vi "parseModeFrame.vi"(8 "error in (no error)":errorcluster, 10 "ModbusBuffer in":refnum<class "ModbusBuffer.lvclass">, 11 "ILC in":refnum<class "ILC.lvclass">) -> (0 "error out":errorcluster, 2 "ModbusBuffer out":refnum<class "ModbusBuffer.lvclass">, 3 "ILC out":refnum<class "ILC.lvclass">)   [LabVIEW 2016, in "RTILC.lvlib" / "ILC.lvclass"]
uses:
  ILC.lvclass
  Common_RT_Modbus/ModbusBuffer/ModbusBuffer.lvclass
  Common_RT_Modbus/ModbusBuffer/ModbusBuffer.lvclass/ModbusBuffer.ctl
  Common_RT_Modbus/DataTypes/ExceptionCodes.ctl
  ILC.lvclass/ILC.ctl
  Common_RT_Modbus/ModbusBuffer/readU8.vi
  Common_RT_Modbus/ModbusBuffer/readTimestampByte.vi
  Common_RT_Modbus/ModbusBuffer/readInstructionByte.vi
  Common_RT_Modbus/RTModbus.lvlib
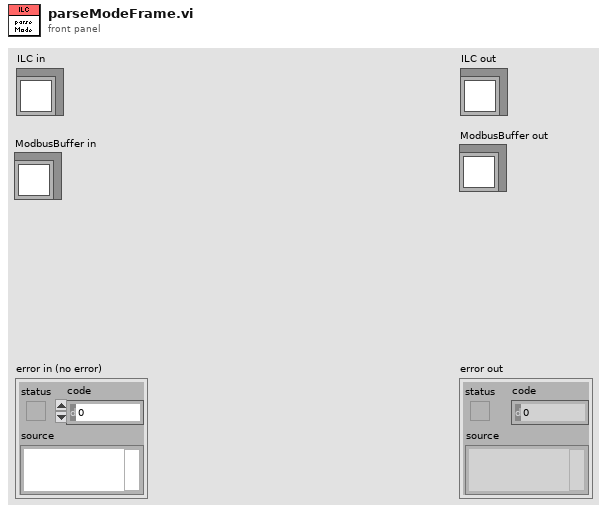
[diagram p1: front panel]
types:
  T1 = typedef "RTModbus.lvlib/ExceptionCodes.ctl" = u16
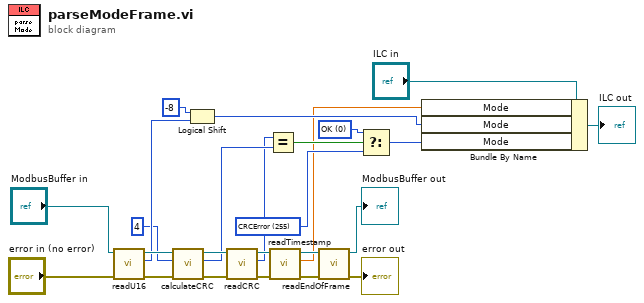
[diagram p0: block diagram]
diagram:
  w21 = T1 255 items=["OK"=0, "IllegalFunction"=1, "IllegalDataAddress"=2, "IllegalDataValue"=3, "SlaveDeviceFailure"=4, "Acknowledge"=5, "SlaveDeviceBusy"=6, "NegativeAcknowledge"=7, "MemoryParityError"=8, "GatewayPathUnavailable"=9, "GatewayTargetDeviceFailedToRespond"=10, "WaitingForResponse"=254, "CRCError"=255] ("f")
  w22 = T1 0 items=["OK"=0, "IllegalFunction"=1, "IllegalDataAddress"=2, "IllegalDataValue"=3, "SlaveDeviceFailure"=4, "Acknowledge"=5, "SlaveDeviceBusy"=6, "NegativeAcknowledge"=7, "MemoryParityError"=8, "GatewayPathUnavailable"=9, "GatewayTargetDeviceFailedToRespond"=10, "WaitingForResponse"=254, "CRCError"=255] ("Responses.ADCOffsetSensitivity")
  n1 = call "readU16.vi"("error in (no error)"="error in (no error)", "ModbusBuffer in"="ModbusBuffer in") -> ("error out"=w7:errorcluster, "Output"=w5:u16, "ModbusBuffer out"=w10:refnum<class "ModbusBuffer.lvclass">)  [unwired: 7 in]
  n2 = call "calculateCRC.vi"("error in (no error)"=w7, "Length"=4, "ModbusBuffer in"=w10) -> ("error out"=w12:errorcluster, "CRC"=w3:u16, "ModbusBuffer out"=w17:refnum<class "ModbusBuffer.lvclass">)  [unwired: 6 in]
  n3 = Logical Shift(y=i16 -8, x=w5) -> (x << y=w18:u16)
  n4 = call "readCRC.vi"("error in (no error)"=w12, "ModbusBuffer in"=w17) -> ("error out"=w13:errorcluster, "Output"=w2:u16, "ModbusBuffer out"=w16:refnum<class "ModbusBuffer.lvclass">)  [unwired: 7 in]
  n5 = Equal?(x=w2, y=w3) -> (x = y?=w23:bool)
  n6 = call "readTimestamp.vi"("error in (no error)"=w13, "ModbusBuffer in"=w16) -> ("error out"=w14:errorcluster, "Output"=w1:dbl, "ModbusBuffer out"=w15:refnum<class "ModbusBuffer.lvclass">)  [unwired: 7 in]
  n7 = call "readEndOfFrame.vi"("error in (no error)"=w14, "ModbusBuffer in"=w15) -> ("error out"=→"error out":errorcluster, "ModbusBuffer out"=→"ModbusBuffer out":refnum<class "ModbusBuffer.lvclass">)  [unwired: 8 in]
  n8 = Select(t=w22, s=w23, f=w21) -> (s? t:f=w19:T1)
  n9 = Bundle By Name(cluster="ILC in", "Mode"=w1, "Mode"=w18, "Mode"=w19) -> (→"ILC out":refnum<class "ILC.lvclass">)
